vi "生成log文件.vi"(3 "error in (no error)":errorcluster, 4 "信息":string, 5 "refnum in":refnum<file>) -> (0 "error out":errorcluster, 1 "String":string, 2 "refnum out":refnum<file>)   [LabVIEW 2013]
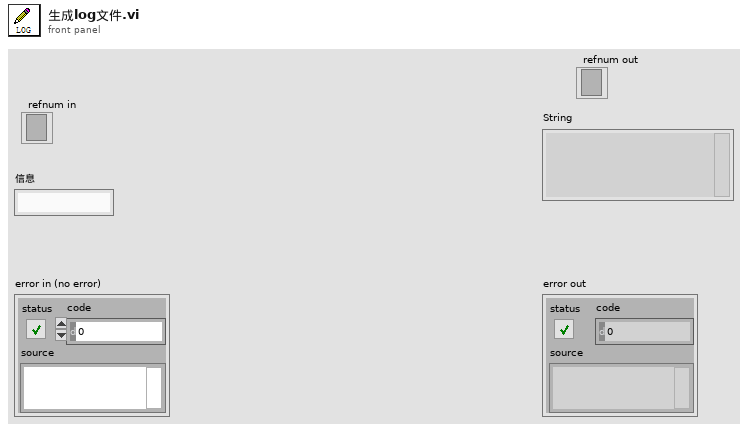
[diagram p1: front panel]
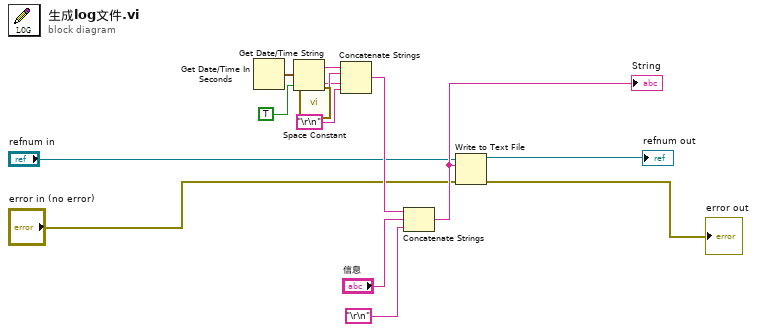
[diagram p0: block diagram]
diagram:
  n1 = Get Date/Time In Seconds() -> (seconds since 1Jan1904=w9:timestamp)
  n2 = Get Date/Time String(seconds (now)=w9, want seconds? (F)=TRUE) -> (date string=w10:string, time string=w12:string)  [unwired: 1 in]
  n3 = call <vilib>:"Space Constant.vi"() -> ("String"=w13:string)
  n4 = Concatenate Strings(w10, w13, w12, "\r\n") -> (w8:string)
  n5 = Concatenate Strings(w8, "信息", "\r\n") -> (w5:string)
  "String" <- w5
  n6 = Write to Text File(file (use dialog)="refnum in", text=w5, error in="error in (no error)") -> (refnum out=→"refnum out":refnum<file>, error out=→"error out":errorcluster)  [unwired: 1 in, 1 out]
